vi "Read from File.vi"(8 "error in":errorcluster, 11 "refnum":refnum<file>) -> (0 "error out":errorcluster, 2 "text":string, 3 "refnum out":refnum<file>)   [LabVIEW 2023]
doc: "Reads the text from the file that the Open File VI opened.\n\nUse this VI as VI under test for Read from File.lvtest."
panel:
  # "Overview: Use this VI as the VI under test for Read from File.lvtest.\nRequirements: LabVIEW Full Development System, Unit Test Framework Toolkit\nInstructions: \n1.  Execute the Read from File.lvtest test file for this VI. In the Project Explorer window, right-click Read from File.lvtest, and select Run from the shortcut menu.\n2.  In the Project Explorer window, double-click Read from File.lvtest to display the Test Properties dialog box.\n3.  Select Setup/Teardown from the Category list to display the Setup/Teardown page. You can understand how LabVIEW passes values among the setup VI, the VI under test, and the teardown VI."
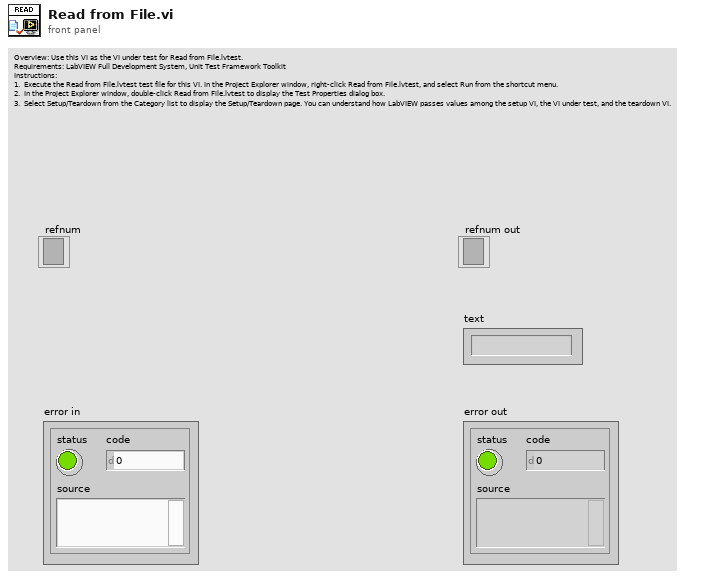
[diagram p1: front panel]
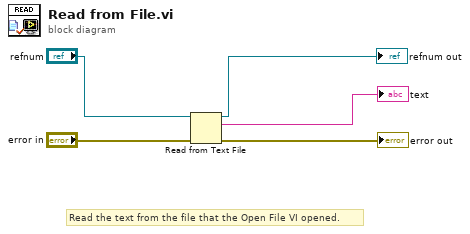
[diagram p0: block diagram]
diagram:
  # "Read the text from the file that the Open File VI opened."
  n1 = Read from Text File(file (use dialog)="refnum", error in="error in") -> (refnum out=→"refnum out":refnum<file>, text=→"text":string, error out=→"error out":errorcluster)  [unwired: 1 in, 2 out]
